vi "slave not available error.vi"(8 "error in":errorcluster, 9 "source":string="slave not available.vi", 11 "slave":i8) -> (0 "error out":errorcluster)   [LabVIEW 2013, in "Profibus Module runtime.lvclass"]
uses:
  Profibus Module runtime.lvclass
  <vilib>/NI/Configuration Framework/NISE_CEF_TreeControl.lvlib
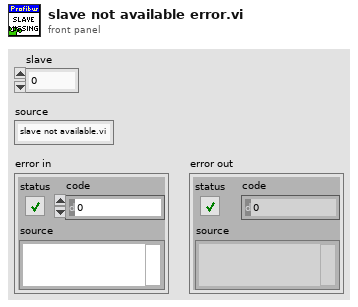
[diagram p1: front panel]
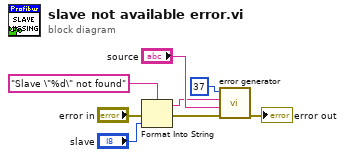
[diagram p0: block diagram]
diagram:
  n1 = Format Into String(format string="Slave \"%d\" not found", error in="error in", "slave") -> (resulting string=w2:string, error out=w4:errorcluster)  [unwired: 1 in]
  n2 = call <vilib>:"error generator.vi"("error in"=w4, "source"="source", "append error message"=w2, "error code (0)"=37) -> ("error out"=→"error out":errorcluster)  [unwired: 5 in]
